vi "listPort.vi"() -> ()   [LabVIEW 2018]
panel:
  in  "串口通信端口":refnum<visa-resource-name>
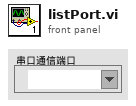
[diagram p1: front panel]
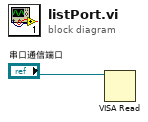
[diagram p0: block diagram]
diagram:
  n1 = VISA Read(VISA resource name="串口通信端口") -> ()  [unwired: 2 in, 4 out]
